vi "Sampler Signals (B).vi"(0 "Sampler":refnum<k24>, 1 "EI":refnum<k24>, 5 "measure":bool, 11 "error in":errorcluster) -> (4 "X":dbl, 6 "Y":dbl, 7 "Signal X":string(combo), 8 "XY Graph":cluster{"Y":dbl[], "Y":dbl[]}[](graph), 9 "Signal Y":string(combo), 10 "PotentialApplied":dbl, 15 "error out":errorcluster)   [LabVIEW 2011]
doc: "Shows the signals from the sampler. The signals are selected with constants. Only for Cyclic Voltammetry measurements. (basic version)"
uses:
  C:/Program Files/Metrohm Autolab/Autolab SDK 1.10/EcoChemie.Autolab.Sdk.dll
  EcoChemie.Autolab.Sdk.dll
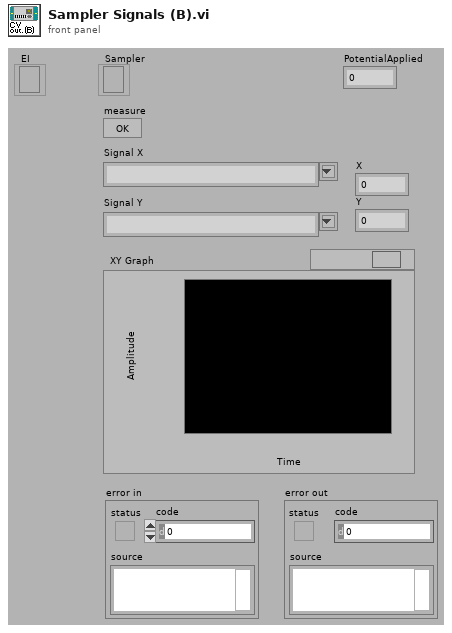
[diagram p1: front panel]
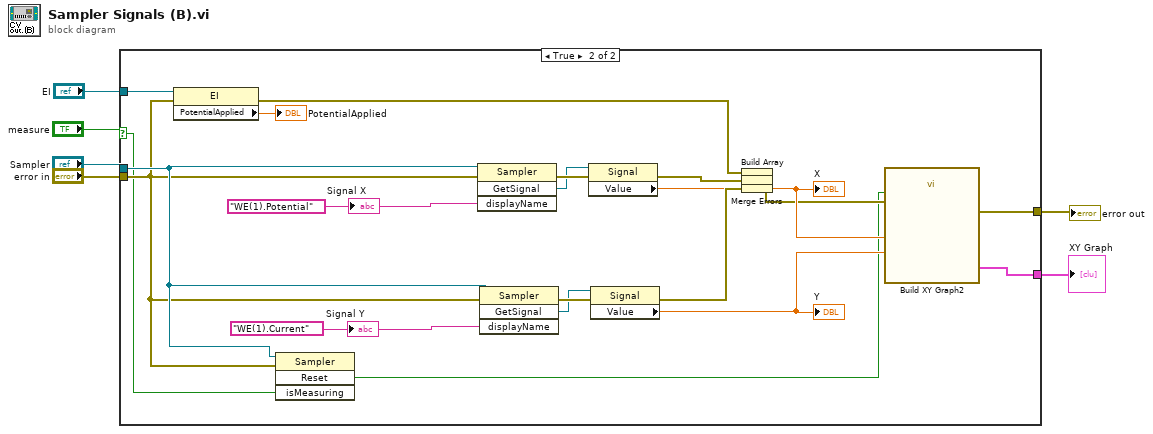
[diagram p0: block diagram]
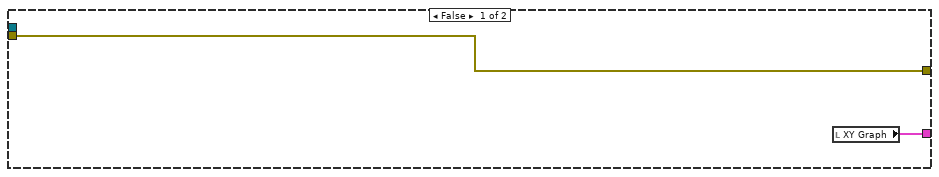
[diagram p2: hidden frame]
diagram:
  n1 = case shown="True" "measure" {
    selector: "measure" -> [_ w11]
    tunnel: [w8 w18] -> w4
    tunnel: "Sampler" -> [_ w13]
    tunnel: "error in" -> [w8 w12]
    tunnel: [w7 w19] -> w5
    tunnel: "EI" -> [_ w16]
    frame False {
      n2 = local read "XY Graph"() -> (w7:cluster{"Y":dbl[], "Y":dbl[]}[])
    }
    frame True {
      w27 = "WE(1).Current" ("Signal Y")
      w28 = "WE(1).Potential" ("Signal X")
      n3 = property class="EI"(reference=w16, error in=w12) -> (error out=w15:errorcluster, "PotentialApplied"=→"PotentialApplied":dbl)  [unwired: 1 out]
      n4 = invoke class="Sampler" method="Reset"(reference=w13, error in=w12, "isMeasuring"=w11) -> ("Reset"=w10:bool)  [unwired: 1 in, 3 out]
      n5 = invoke class="Sampler" method="GetSignal"(reference=w13, error in=w12, "displayName"=w28) -> (error out=w26:errorcluster, "GetSignal"=w24:refnum<k24>)  [unwired: 1 in, 2 out]
      n6 = invoke class="Sampler" method="GetSignal"(reference=w13, error in=w12, "displayName"=w27) -> (error out=w25:errorcluster, "GetSignal"=w23:refnum<k24>)  [unwired: 1 in, 2 out]
      n7 = property class="Signal"(reference=w24, error in=w26) -> (error out=w14:errorcluster, "Value"=w21:dbl)  [unwired: 1 out]
      "X" <- w21
      n8 = property class="Signal"(reference=w23, error in=w25) -> (error out=w29:errorcluster, "Value"=w22:dbl)  [unwired: 1 out]
      "Y" <- w22
      n9 = Build Array(w15, w14, w29) -> (w9:errorcluster[])
      n10 = Merge Errors(w9) -> (w20:errorcluster)
      n11 = call "Build XY Graph2"("error in (no error)"=w20, "Reset"=w10, "Y Input"=w22, "X Input"=w21) -> ("error out"=w18:errorcluster, "XY Graph"=w19:cluster{"Y":dbl[], "Y":dbl[]}[])  [unwired: 6 in]
      "Signal X" <- w28
      "Signal Y" <- w27
    }
  }
  "error out" <- w4
  "XY Graph" <- w5
